vi "Write Nickname.vi"(8 "error in (no error)":errorcluster, 10 "Nickname":string, 11 "Bill Murray in":refnum<class "Bill Murray.lvclass">) -> (0 "error out":errorcluster, 3 "Bill Murray out":refnum<class "Bill Murray.lvclass">)   [LabVIEW 2019, in "Bill Murray.lvclass"]
uses:
  Bill Murray.lvclass
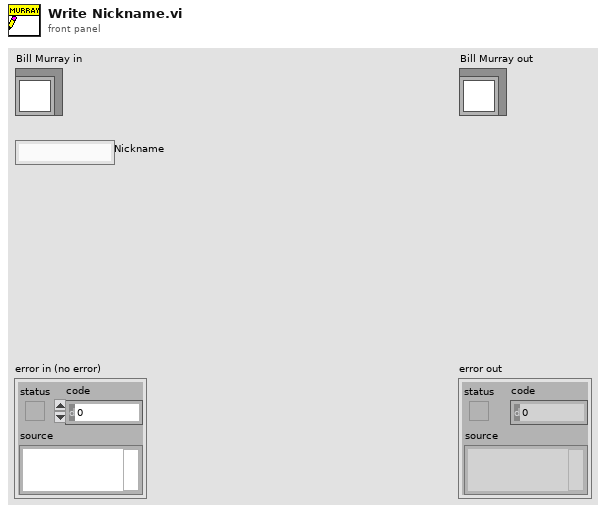
[diagram p1: front panel]
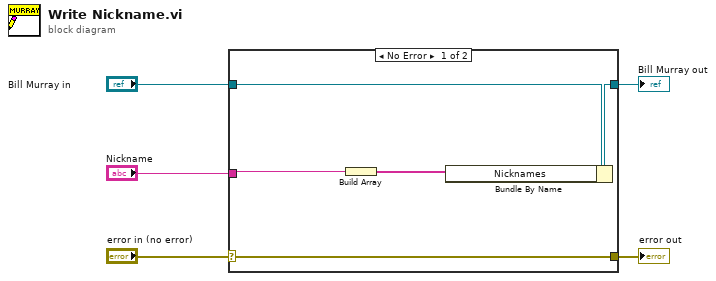
[diagram p0: block diagram]
diagram:
  n1 = case shown="No Error" "error in (no error)" {
    selector: "error in (no error)" -> [w10 w11]
    tunnel: [w10 w11] -> w4
    tunnel: [w8 w12] -> w2
    tunnel: "Bill Murray in" -> [w9 w12]
    tunnel: "Nickname" -> [w7 _]
    frame No Error {
      n2 = Build Array(w7) -> (w6:string[])
      n3 = Bundle By Name(cluster=w9, "Nicknames"=w6) -> (w8:refnum<class "Bill Murray.lvclass">)
    }
    frame Error {
    }
  }
  "error out" <- w4
  "Bill Murray out" <- w2
